vi "initializeRobcomm.vi"(2 "error in":errorcluster, 3 "close serial":bool, 4 "timeout (sec)":u32=1, 5 "VISA resource name":refnum<visa-resource-name>="COM1") -> (0 "error out":errorcluster, 1 "serial out":refnum<visa-resource-name>="COM1")   [LabVIEW 2012]
uses:
  serialTypeDef.ctl
  <vilib>/Instr/_visa.llb/VISA Open Access Mode.ctl
  <vilib>/Instr/_visa.llb/VISA Configure Serial Port (Instr).vi
panel:
  out "read buffer":string
  out "no echo readout":string
  out "HC":u32
  out "ENQS":string
  out "Curr State":T1=enum."ack2"
  out "TIORC2":u32
  out "TIORC1":u32
  out "Prev State":T1=enum."ack2"
  out "NHRS":string
  out "NHRC":u32
  out "NERC":u32
  out "TIORS1":string
  out "TIORS2":string
  out "loop catch":i32
  out "ETXRS":string
  # "final out should look like:\n\n\"\n>>\""
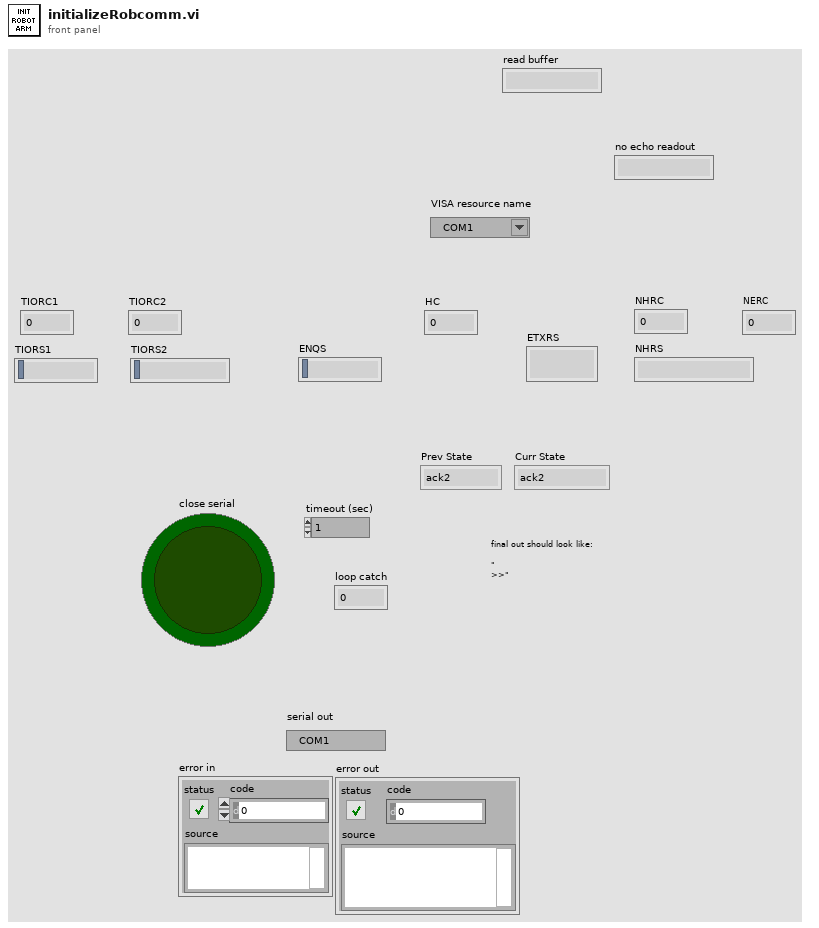
[diagram p1: front panel]
types:
  T1 = typedef "serialTypeDef.ctl" = enum16{"test if open", "open serial", "enquiry seq", "header seq", "ack1", "ack2", "etx", "no help", "no echo", "end", "close serial", "nothing"}
  T2 = typedef "VISA Open Access Mode.ctl" = u32
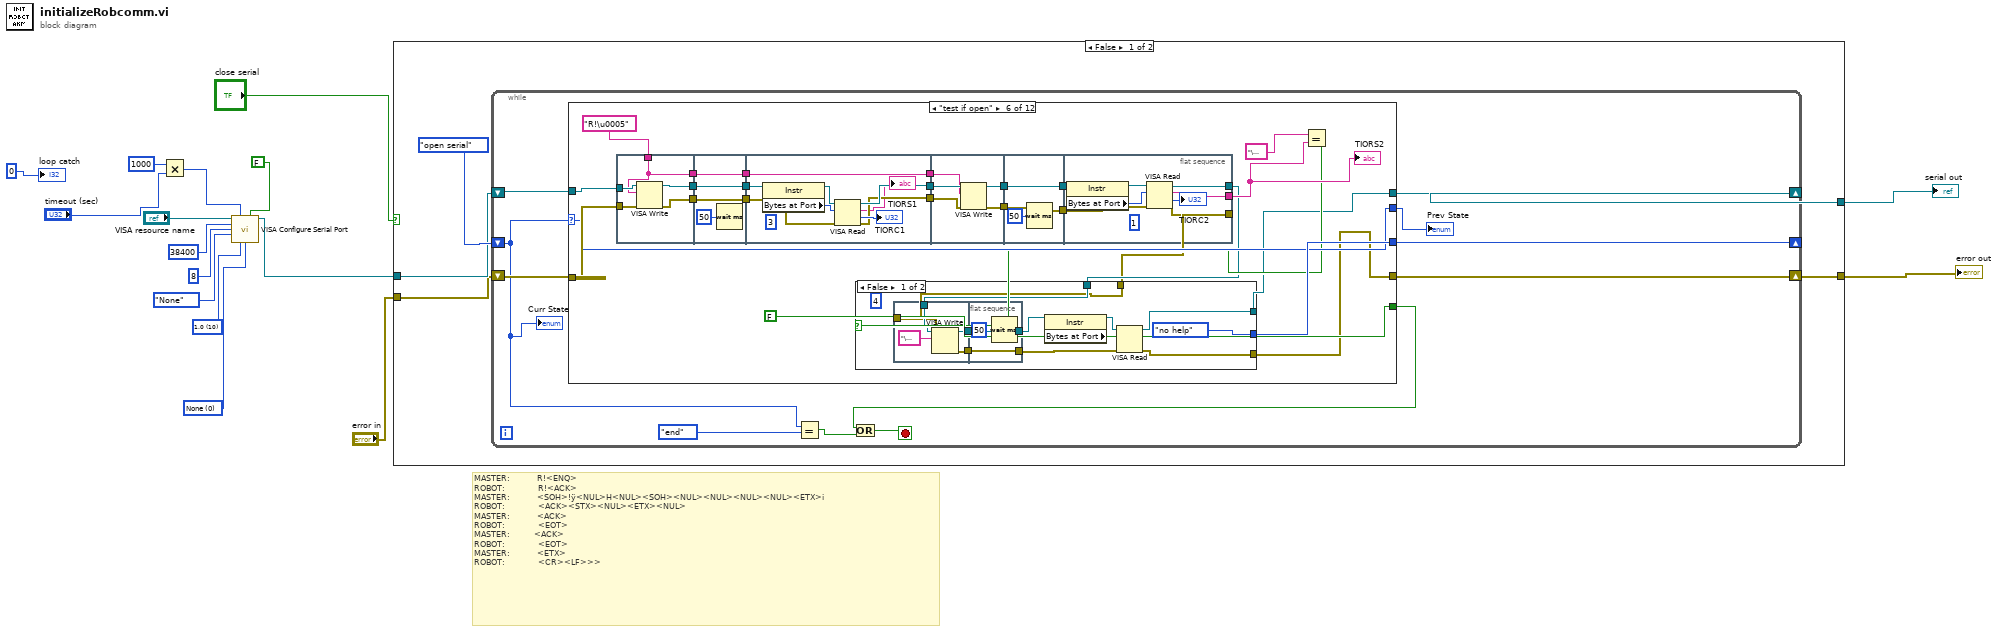
[diagram p0: block diagram]
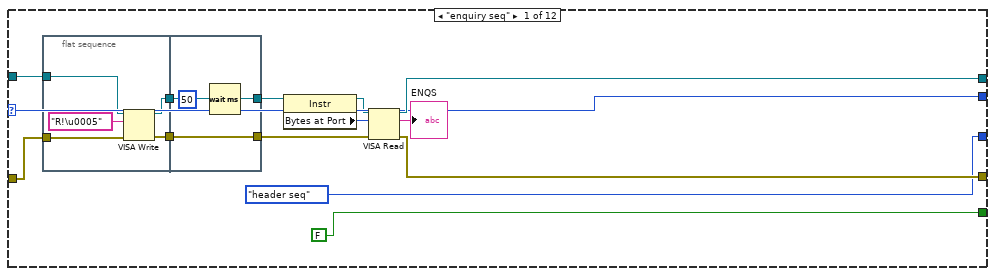
[diagram p2: hidden frame]
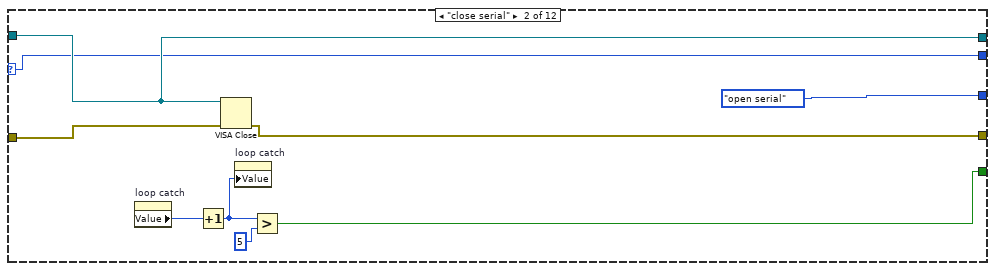
[diagram p3: hidden frame]
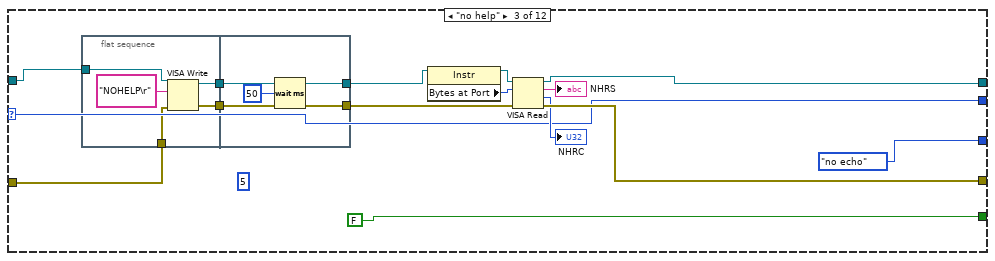
[diagram p4: hidden frame]
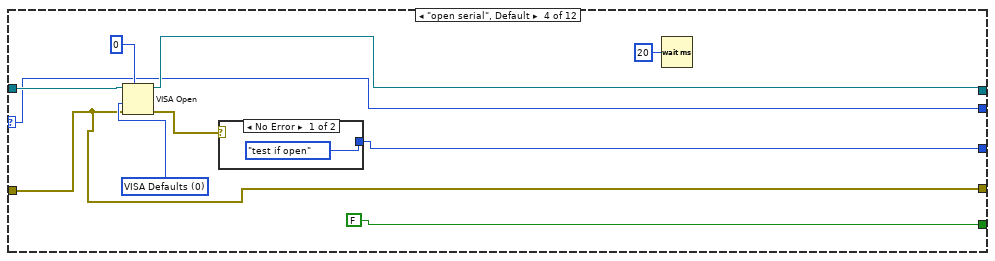
[diagram p5: hidden frame]
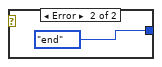
[diagram p6: hidden frame]
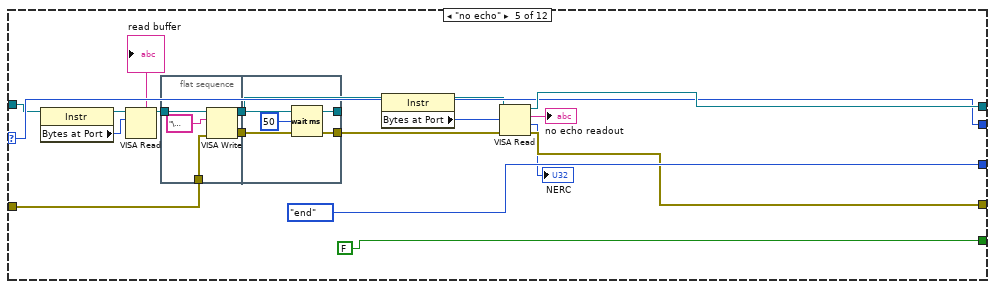
[diagram p7: hidden frame]
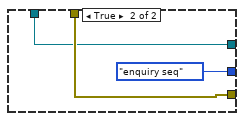
[diagram p8: hidden frame]
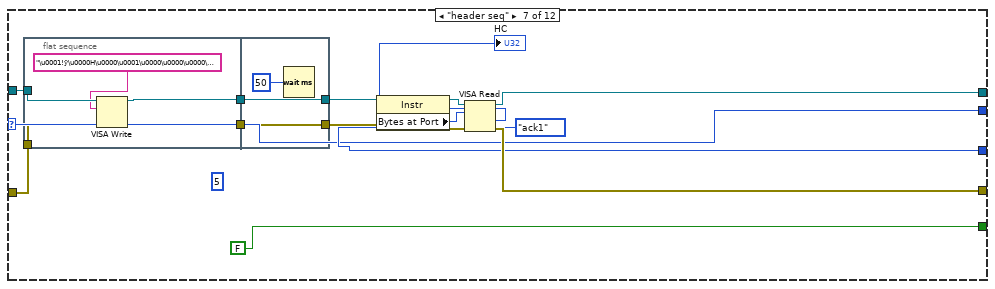
[diagram p9: hidden frame]
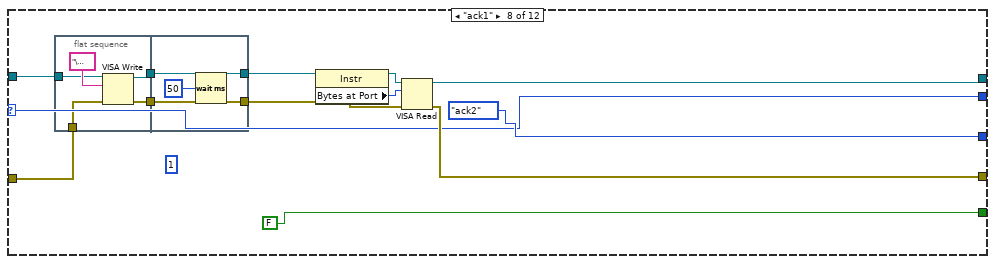
[diagram p10: hidden frame]
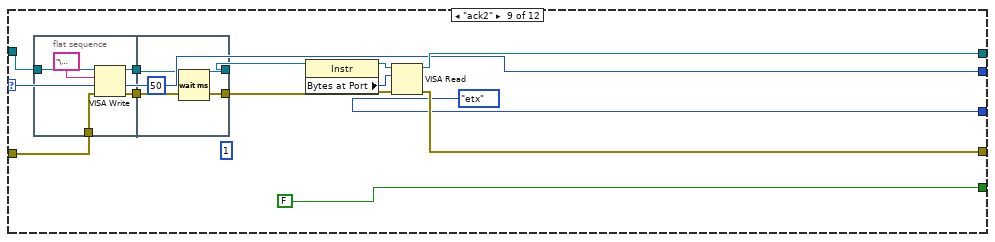
[diagram p11: hidden frame]
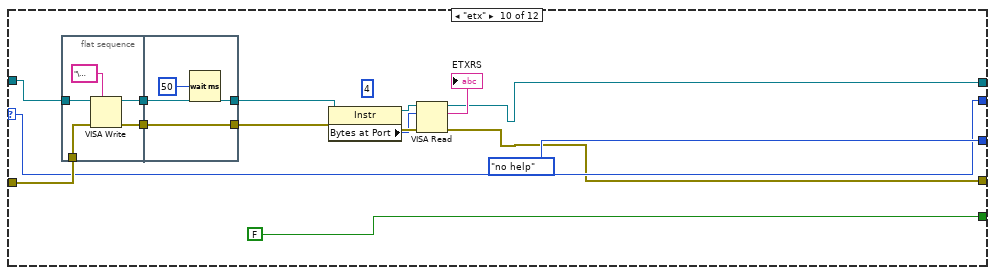
[diagram p12: hidden frame]
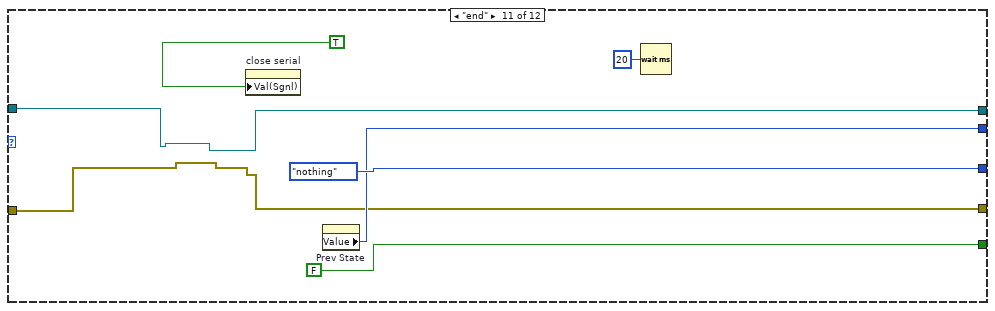
[diagram p13: hidden frame]
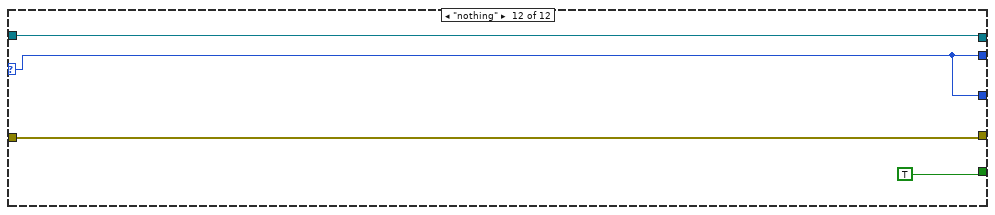
[diagram p14: hidden frame]
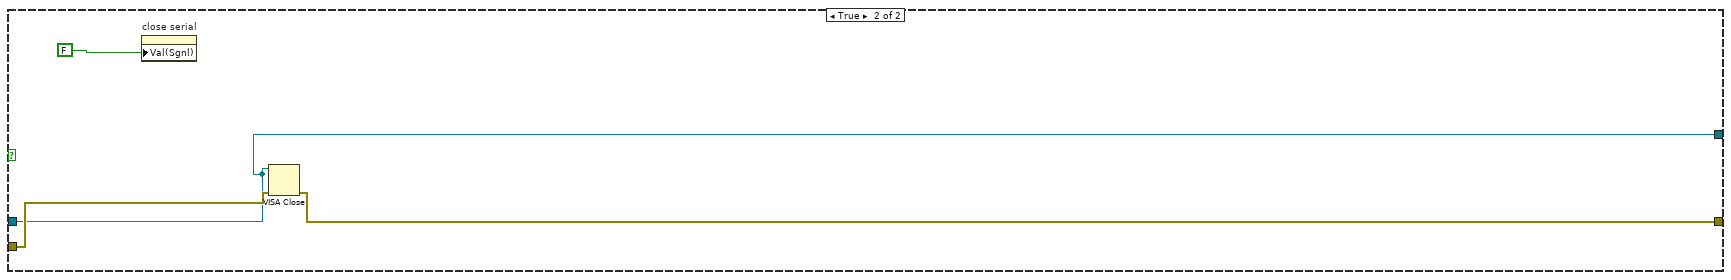
[diagram p15: hidden frame]
diagram:
  w6 = u16 0 items=["None", "XON/XOFF", "RTS/CTS", "XON/XOFF & RTS/CTS", "DTR/DSR", "XON/XOFF & DTR/DSR"] ("flow control (0:none)")
  w5 = u16 10 items=["1.0"=10, "1.5"=15, "2.0"=20] ("stop bits (10: 1 bit)")
  # "MASTER:         R!<ENQ>\nROBOT:           R!<ACK>\nMASTER:         <SOH>!ÿ<NUL>H<NUL><SOH><NUL><NUL><NUL><NUL><ETX>i\nROBOT:           <ACK><STX><NUL><ETX><NUL>\nMASTER:         <ACK>\nROBOT:           <EOT>\nMASTER:        <ACK>\nROBOT:           <EOT>\nMASTER:         <ETX>\nROBOT:           <CR><LF>>>"
  n1 = Multiply(x=u32 1000, y="timeout (sec)") -> (x*y=w10:u32)
  n2 = call-poly "VISA Configure Serial Port"("VISA resource name"="VISA resource name", "timeout (10sec)"=w10, "Enable Termination\nChar (T)"=FALSE ("Enable Termination\nChar (T)"), "baud rate (9600)"=u32 38400, "data bits (8)"=u16 8, "parity (0:none)"=enum16{"None", "Odd", "Even", "Mark", "Space"}."None", "stop bits (10: 1 bit)"=w5, "flow control (0:none)"=w6) -> ("VISA resource name out"=w1:refnum<visa-resource-name>)  [unwired: 6 in, 1 out]
  n3 = case shown="False" "close serial" {
    tunnel: [w21 w307] -> w16
    tunnel: [w20 w306] -> w15
    tunnel: w1 -> [w18 w306]
    tunnel: "error in" -> [w17 w308]
    frame False {
      n4 = while {
        shift-right: [w31] -> w20
        shift-left: w18 -> [w32]
        shift-right: [w29] -> w21
        shift-left: w17 -> [w30]
        shift-right: [w24] -> _
        shift-left: serialTypeDef."open serial" -> [w23]
        stop <- w25 stop-if-true
        n5 = case shown="\"test if open\"" w23 {
          selector: w23 -> [w39 w56 w69 w88 w110 w147 w214 w236 w256 w279 _ w303]
          tunnel: w32 -> [w46 w63 w78 w95 w108 w150 w221 w234 w263 w285 w296 w304]
          tunnel: [w42 w63 w73 w93 w113 w128 w220 w242 w259 w273 w296 w304] -> w31
          tunnel: w30 -> [w45 w62 w77 w91 w116 w149 w218 w241 w262 w284 w295 w302]
          tunnel: [w43 w61 w75 w91 w112 w127 w219 w239 w260 w272 w295 w302] -> w29
          tunnel: [serialTypeDef."header seq" serialTypeDef."open serial" serialTypeDef."no echo" w90 serialTypeDef."end" w151 serialTypeDef."ack1" serialTypeDef."ack2" serialTypeDef."etx" serialTypeDef."no help" serialTypeDef."nothing" w303] -> w24
          tunnel: [FALSE w57 FALSE FALSE FALSE FALSE FALSE FALSE FALSE FALSE FALSE TRUE] -> w27
          tunnel: [w39 w56 w69 w88 w110 w147 w214 w236 w256 w279 w297 w303] -> w22
          frame "enquiry seq" {
            n6 = flat-sequence {
              tunnel: w46 -> [w50]
              tunnel: w45 -> [w49]
              tunnel: [w48] -> w34
              tunnel: [w47] -> w33
              tunnel: [w53] -> w36
              tunnel: [w54] -> w44
              tunnel: w34 -> [w54]
              tunnel: w33 -> [w53]
              frame #0 {
                n7 = VISA Write(VISA resource name=w50, write buffer="R!\u0005", error in (no error)=w49) -> (VISA resource name out=w47:refnum<visa-resource-name>, error out=w48:errorcluster)  [unwired: 1 out]
              }
              frame #1 {
                n8 = Wait (ms)(milliseconds to wait=u32 50) -> ()  [unwired: 1 out]
              }
            }
            n9 = property class="Instr"(reference=w36) -> (reference out=w35:refnum<visa-resource-name>, "Bytes at Port"=w37:u32)  [unwired: 1 in, 1 out]
            n10 = VISA Read(VISA resource name=w35, byte count=w37, error in (no error)=w44) -> (VISA resource name out=w42:refnum<visa-resource-name>, read buffer=→"ENQS":string, error out=w43:errorcluster)  [unwired: 1 out]
          }
          frame "close serial" {
            n11 = property on="loop catch" class="DigNum (strict)"() -> ("Value"=w60:i32)  [unwired: 2 in, 2 out]
            n12 = Increment(x=w60) -> (x+1=w59:i32)
            n13 = VISA Close(VISA resource name=w63, error in (no error)=w62) -> (error out=w61:errorcluster)
            n14 = property on="loop catch" class="DigNum (strict)"("Value"=w59) -> ()  [unwired: 2 in, 2 out]
            n15 = Greater?(x=w59, y=5) -> (0:w57:bool)
          }
          frame "no help" {
            (unwired) 5
            n16 = flat-sequence {
              tunnel: w78 -> [w83]
              tunnel: w77 -> [w82]
              tunnel: [w81] -> w65
              tunnel: [w79] -> w64
              tunnel: [w85] -> w68
              tunnel: [w86] -> w76
              tunnel: w65 -> [w86]
              tunnel: w64 -> [w85]
              frame #0 {
                n17 = VISA Write(VISA resource name=w83, write buffer="NOHELP\r", error in (no error)=w82) -> (VISA resource name out=w79:refnum<visa-resource-name>, error out=w81:errorcluster)  [unwired: 1 out]
              }
              frame #1 {
                n18 = Wait (ms)(milliseconds to wait=u32 50) -> ()  [unwired: 1 out]
              }
            }
            n19 = property class="Instr"(reference=w68) -> (reference out=w67:refnum<visa-resource-name>, "Bytes at Port"=w66:u32)  [unwired: 1 in, 1 out]
            n20 = VISA Read(VISA resource name=w67, byte count=w66, error in (no error)=w76) -> (VISA resource name out=w73:refnum<visa-resource-name>, read buffer=→"NHRS":string, return count=→"NHRC":u32, error out=w75:errorcluster)
          }
          frame "open serial", Default {
            w94 = T2 0 items=["VISA Defaults"=0, "Exclusive Lock"=1, "Load Configured Settings"=4] ("Access Mode")
            n21 = VISA Open(timeout (0)=u32 0 ("VISA Open timeout (0)"), access mode=w94, error in (no error)=w91, VISA resource name=w95) -> (VISA resource name=w93:refnum<visa-resource-name>, error out=w92:errorcluster)  [unwired: 1 in]
            n22 = case shown="No Error" w92 {
              tunnel: [serialTypeDef."test if open" serialTypeDef."end"] -> w90
              frame No Error {
              }
              frame Error {
              }
            }
            n23 = Wait (ms)(milliseconds to wait=u32 20) -> ()  [unwired: 1 out]
          }
          frame "no echo" {
            n24 = property class="Instr"(reference=w108) -> (reference out=w106:refnum<visa-resource-name>, "Bytes at Port"=w107:u32)  [unwired: 1 in, 1 out]
            n25 = VISA Read(VISA resource name=w106, byte count=w107) -> (VISA resource name out=w105:refnum<visa-resource-name>, read buffer=→"read buffer":string)  [unwired: 1 in, 2 out]
            n26 = flat-sequence {
              tunnel: w116 -> [w121]
              tunnel: w105 -> [w119]
              tunnel: [w120] -> w100
              tunnel: [w118] -> w99
              tunnel: [w124] -> w103
              tunnel: [w125] -> w114
              tunnel: w100 -> [w125]
              tunnel: w99 -> [w124]
              frame #0 {
                n27 = VISA Write(VISA resource name=w119, write buffer="\u0012", error in (no error)=w121) -> (VISA resource name out=w118:refnum<visa-resource-name>, error out=w120:errorcluster)  [unwired: 1 out]
              }
              frame #1 {
                n28 = Wait (ms)(milliseconds to wait=u32 50) -> ()  [unwired: 1 out]
              }
            }
            n29 = property class="Instr"(reference=w103) -> (reference out=w102:refnum<visa-resource-name>, "Bytes at Port"=w104:u32)  [unwired: 1 in, 1 out]
            n30 = VISA Read(VISA resource name=w102, byte count=w104, error in (no error)=w114) -> (VISA resource name out=w113:refnum<visa-resource-name>, read buffer=→"no echo readout":string, return count=→"NERC":u32, error out=w112:errorcluster)
          }
          frame "test if open" {
            n31 = flat-sequence {
              tunnel: w150 -> [w156]
              tunnel: w149 -> [w155]
              tunnel: [w154] -> w146
              tunnel: "R!\u0005" -> [w153]
              tunnel: [w153] -> w140
              tunnel: [w152] -> w134
              tunnel: w146 -> [w159]
              tunnel: [w159] -> w145
              tunnel: [w158] -> w141
              tunnel: w140 -> [w158]
              tunnel: w134 -> [w157]
              tunnel: [w157] -> w133
              tunnel: w145 -> [w163]
              tunnel: [w169] -> w144
              tunnel: [w168] -> w142
              tunnel: w141 -> [w168]
              tunnel: [w166] -> w135
              tunnel: w133 -> [w165]
              tunnel: w144 -> [w174]
              tunnel: w142 -> [w172]
              tunnel: [w173] -> w139
              tunnel: [w171] -> w137
              tunnel: w135 -> [w170]
              tunnel: w139 -> [w177]
              tunnel: [w177] -> w138
              tunnel: w137 -> [w175]
              tunnel: [w175] -> w136
              tunnel: [w185] -> w129
              tunnel: w138 -> [w180]
              tunnel: [w184] -> w131
              tunnel: [w183] -> w126
              tunnel: w136 -> [w182]
              frame #0 {
                n32 = VISA Write(VISA resource name=w156, write buffer=w153, error in (no error)=w155) -> (VISA resource name out=w154:refnum<visa-resource-name>, error out=w152:errorcluster)  [unwired: 1 out]
              }
              frame #1 {
                n33 = Wait (ms)(milliseconds to wait=u32 50) -> ()  [unwired: 1 out]
              }
              frame #2 {
                (unwired) u32 3 ("milliseconds to wait")
                n34 = property class="Instr"(reference=w163) -> (reference out=w161:refnum<visa-resource-name>, "Bytes at Port"=w162:u32)  [unwired: 1 in, 1 out]
                n35 = VISA Read(VISA resource name=w161, byte count=w162, error in (no error)=w165) -> (VISA resource name out=w169:refnum<visa-resource-name>, read buffer=→"TIORS1":string, return count=→"TIORC1":u32, error out=w166:errorcluster)
              }
              frame #3 {
                n36 = VISA Write(VISA resource name=w174, write buffer=w172, error in (no error)=w170) -> (VISA resource name out=w173:refnum<visa-resource-name>, error out=w171:errorcluster)  [unwired: 1 out]
              }
              frame #4 {
                n37 = Wait (ms)(milliseconds to wait=u32 50) -> ()  [unwired: 1 out]
              }
              frame #5 {
                (unwired) u32 1 ("milliseconds to wait")
                n38 = property class="Instr"(reference=w180) -> (reference out=w179:refnum<visa-resource-name>, "Bytes at Port"=w178:u32)  [unwired: 1 in, 1 out]
                n39 = VISA Read(VISA resource name=w179, byte count=w178, error in (no error)=w182) -> (VISA resource name out=w185:refnum<visa-resource-name>, read buffer=w184:string, return count=→"TIORC2":u32, error out=w183:errorcluster)
              }
            }
            n40 = Equal?(x="\u0004" ("read buffer"), y=w131) -> (x = y?=w130:bool)
            n41 = case shown="False" w130 {
              tunnel: [serialTypeDef."no help" serialTypeDef."enquiry seq"] -> w151
              tunnel: w129 -> [w195 w205]
              tunnel: [w192 w205] -> w128
              tunnel: [w193 w206] -> w127
              tunnel: w126 -> [w186 w206]
              frame False {
                (unwired) u32 4 ("milliseconds to wait")
                n42 = flat-sequence {
                  tunnel: w195 -> [w201]
                  tunnel: [w199] -> w188
                  tunnel: [w198] -> w187
                  tunnel: w186 -> [w197]
                  tunnel: [w203] -> w191
                  tunnel: [w204] -> w194
                  tunnel: w188 -> [w204]
                  tunnel: w187 -> [w203]
                  frame #0 {
                    n43 = VISA Write(VISA resource name=w201, write buffer="\u0003", error in (no error)=w197) -> (VISA resource name out=w198:refnum<visa-resource-name>, error out=w199:errorcluster)  [unwired: 1 out]
                  }
                  frame #1 {
                    n44 = Wait (ms)(milliseconds to wait=u32 50) -> ()  [unwired: 1 out]
                  }
                }
                n45 = property class="Instr"(reference=w191) -> (reference out=w190:refnum<visa-resource-name>, "Bytes at Port"=w189:u32)  [unwired: 1 in, 1 out]
                n46 = VISA Read(VISA resource name=w190, byte count=w189, error in (no error)=w194) -> (VISA resource name out=w192:refnum<visa-resource-name>, error out=w193:errorcluster)  [unwired: 2 out]
              }
              frame True {
              }
            }
            "TIORS2" <- w131
          }
          frame "header seq" {
            (unwired) u32 5 ("byte count")
            n47 = flat-sequence {
              tunnel: w221 -> [w226]
              tunnel: w218 -> [w225]
              tunnel: [w223] -> w209
              tunnel: [w222] -> w208
              tunnel: [w228] -> w210
              tunnel: [w229] -> w217
              tunnel: w209 -> [w229]
              tunnel: w208 -> [w228]
              frame #0 {
                n48 = VISA Write(VISA resource name=w226, write buffer="\u0001!ÿ\u0000H\u0000\u0001\u0000\u0000\u0000\u0000\u0003i" ("write buffer 2"), error in (no error)=w225) -> (VISA resource name out=w222:refnum<visa-resource-name>, error out=w223:errorcluster)  [unwired: 1 out]
              }
              frame #1 {
                n49 = Wait (ms)(milliseconds to wait=u32 50) -> ()  [unwired: 1 out]
              }
            }
            n50 = property class="Instr"(reference=w210) -> (reference out=w211:refnum<visa-resource-name>, "Bytes at Port"=w212:u32)  [unwired: 1 in, 1 out]
            n51 = VISA Read(VISA resource name=w211, byte count=w212, error in (no error)=w217) -> (VISA resource name out=w220:refnum<visa-resource-name>, return count=→"HC":u32, error out=w219:errorcluster)  [unwired: 1 out]
          }
          frame "ack1" {
            (unwired) u32 1 ("byte count")
            n52 = flat-sequence {
              tunnel: w241 -> [w247]
              tunnel: w234 -> [w243]
              tunnel: [w246] -> w231
              tunnel: [w244] -> w230
              tunnel: [w249] -> w235
              tunnel: [w250] -> w240
              tunnel: w231 -> [w250]
              tunnel: w230 -> [w249]
              frame #0 {
                n53 = VISA Write(VISA resource name=w243, write buffer="\u0006", error in (no error)=w247) -> (VISA resource name out=w244:refnum<visa-resource-name>, error out=w246:errorcluster)  [unwired: 1 out]
              }
              frame #1 {
                n54 = Wait (ms)(milliseconds to wait=u32 50) -> ()  [unwired: 1 out]
              }
            }
            n55 = property class="Instr"(reference=w235) -> (reference out=w233:refnum<visa-resource-name>, "Bytes at Port"=w232:u32)  [unwired: 1 in, 1 out]
            n56 = VISA Read(VISA resource name=w233, byte count=w232, error in (no error)=w240) -> (VISA resource name out=w242:refnum<visa-resource-name>, error out=w239:errorcluster)  [unwired: 2 out]
          }
          frame "ack2" {
            (unwired) u32 1 ("byte count")
            n57 = flat-sequence {
              tunnel: w263 -> [w268]
              tunnel: w262 -> [w267]
              tunnel: [w266] -> w252
              tunnel: [w264] -> w251
              tunnel: [w270] -> w253
              tunnel: [w271] -> w261
              tunnel: w252 -> [w271]
              tunnel: w251 -> [w270]
              frame #0 {
                n58 = VISA Write(VISA resource name=w268, write buffer="\u0006", error in (no error)=w267) -> (VISA resource name out=w264:refnum<visa-resource-name>, error out=w266:errorcluster)  [unwired: 1 out]
              }
              frame #1 {
                n59 = Wait (ms)(milliseconds to wait=u32 50) -> ()  [unwired: 1 out]
              }
            }
            n60 = property class="Instr"(reference=w253) -> (reference out=w254:refnum<visa-resource-name>, "Bytes at Port"=w255:u32)  [unwired: 1 in, 1 out]
            n61 = VISA Read(VISA resource name=w254, byte count=w255, error in (no error)=w261) -> (VISA resource name out=w259:refnum<visa-resource-name>, error out=w260:errorcluster)  [unwired: 2 out]
          }
          frame "etx" {
            (unwired) u32 4 ("byte count")
            n62 = flat-sequence {
              tunnel: w285 -> [w290]
              tunnel: w284 -> [w289]
              tunnel: [w288] -> w275
              tunnel: [w286] -> w274
              tunnel: [w292] -> w276
              tunnel: [w293] -> w283
              tunnel: w275 -> [w293]
              tunnel: w274 -> [w292]
              frame #0 {
                n63 = VISA Write(VISA resource name=w290, write buffer="\u0003", error in (no error)=w289) -> (VISA resource name out=w286:refnum<visa-resource-name>, error out=w288:errorcluster)  [unwired: 1 out]
              }
              frame #1 {
                n64 = Wait (ms)(milliseconds to wait=u32 50) -> ()  [unwired: 1 out]
              }
            }
            n65 = property class="Instr"(reference=w276) -> (reference out=w277:refnum<visa-resource-name>, "Bytes at Port"=w278:u32)  [unwired: 1 in, 1 out]
            n66 = VISA Read(VISA resource name=w277, byte count=w278, error in (no error)=w283) -> (VISA resource name out=w273:refnum<visa-resource-name>, read buffer=→"ETXRS":string, error out=w272:errorcluster)  [unwired: 1 out]
          }
          frame "end" {
            n67 = property on="close serial" class="Bool (strict)"("Val(Sgnl)"=TRUE) -> ()  [unwired: 2 in, 2 out]
            n68 = property on="Prev State" class="Enum (strict)"() -> ("Value"=w297:T1)  [unwired: 2 in, 2 out]
            n69 = Wait (ms)(milliseconds to wait=u32 20) -> ()  [unwired: 1 out]
          }
          frame "nothing" {
          }
        }
        "Prev State" <- w22
        n70 = Equal?(x=w23, y=serialTypeDef."end") -> (x = y?=w26:bool)
        n71 = Or(x=w27, y=w26) -> (x .or. y?=w25:bool)
        "Curr State" <- w23
      }
    }
    frame True {
      n72 = property on="close serial" class="Bool (strict)"("Val(Sgnl)"=FALSE) -> ()  [unwired: 2 in, 2 out]
      n73 = VISA Close(VISA resource name=w306, error in (no error)=w308) -> (error out=w307:errorcluster)
    }
  }
  "error out" <- w16
  "serial out" <- w15
  "loop catch" <- 0
